vi "Untitled 5.vi"() -> ()   [LabVIEW 2021]
panel:
  out "output array":dbl[](array[numeric])
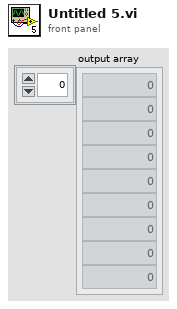
[diagram p1: front panel]
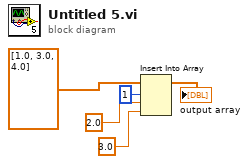
[diagram p0: block diagram]
diagram:
  n1 = Insert Into Array(array=dbl[] [1.0, 3.0, 4.0], index=1, new element #1=2.0 ("new element/subarray"), new element #2=3.0 ("new element/subarray")) -> (→"output array":dbl[])
